vi "Do.vi"(8 "error in (no error)":errorcluster, 10 "Actor in":refnum<class "Actor.lvclass">, 11 "Reset Power Msg":refnum<class "Reset Power Msg.lvclass">) -> (0 "error out":errorcluster, 2 "Actor out":refnum<class "Actor.lvclass">)   [LabVIEW 2018, in "Laser.lvlib" / "Reset Power Msg.lvclass"]
doc: "This VI delivers the message to the actor by calling the appropriate method(s) on the actor."
uses:
  Reset Power Msg.lvclass
  <vilib>/ActorFramework/Actor/Actor.lvclass
  Laser/Laser.lvclass
  C:/Program Files/National Instruments/LabVIEW 2018/vi.lib/ActorFramework/Actor/Actor.lvclass
  Reset Power Msg.lvclass/Reset Power Msg.ctl
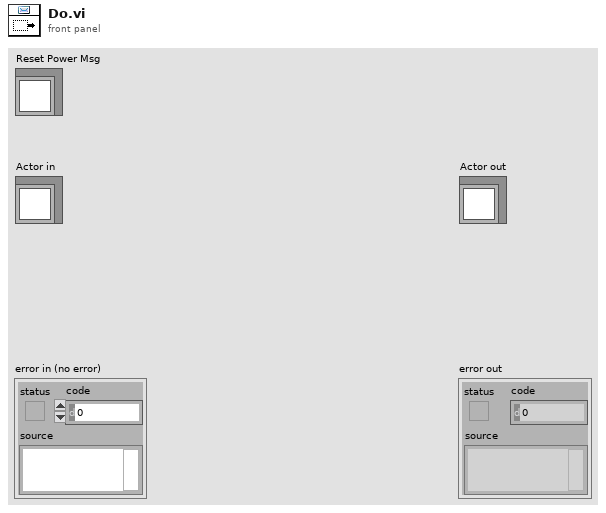
[diagram p1: front panel]
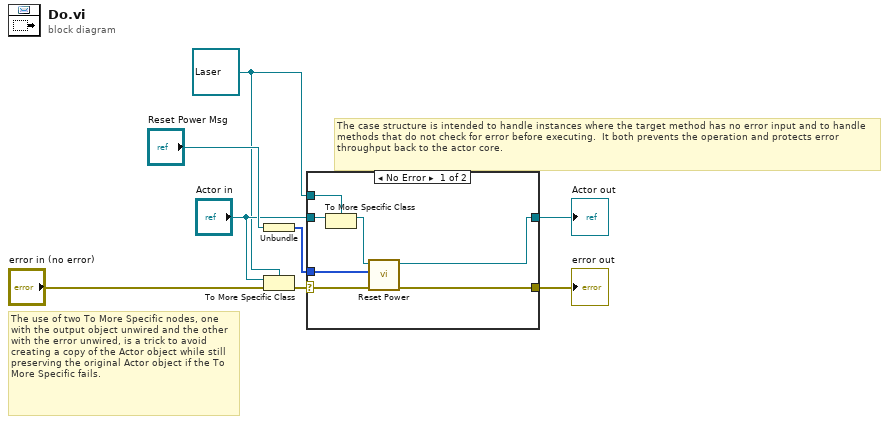
[diagram p0: block diagram]
diagram:
  w2 = refnum<class "Laser.lvclass"> refnum ("Actor in")
  # "The use of two To More Specific nodes, one with the output object unwired and the other with the error unwired, is a trick to avoid creating a copy of the Actor object while still preserving the original Actor object if the To More Specific fails."
  # "The case structure is intended to handle instances where the target method has no error input and to handle methods that do not check for error before executing.  It both prevents the operation and protects error throughput back to the actor core."
  n1 = Unbundle("Reset Power Msg") -> (w1:u16[])
  n2 = To More Specific Class(target class=w2, reference="Actor in", error in="error in (no error)") -> (error out=w6:errorcluster)  [unwired: 1 out]
  n3 = case shown="No Error" w6 {
    selector: w6 -> [w13 w17]
    tunnel: [w15 w17] -> w5
    tunnel: [w14 w16] -> w4
    tunnel: "Actor in" -> [w12 w16]
    tunnel: w2 -> [w11 _]
    tunnel: w1 -> [w9 _]
    frame No Error {
      n4 = To More Specific Class(target class=w11, reference=w12) -> (specific class reference=w10:refnum<class "Laser.lvclass">)  [unwired: 1 in, 1 out]
      n5 = call-dynamic "Reset Power.vi"("error in (no error)"=w13, "Wavelengths"=w9, "Laser in"=w10) -> ("error out"=w15:errorcluster, "Laser out"=w14:refnum<class "Laser.lvclass">)  [unwired: 7 in]
    }
    frame Error {
      # "If type check fails, pass the original object out again."
    }
  }
  "error out" <- w5
  "Actor out" <- w4
